vi "ProjectPaths.vi"(7 "Item":T1, 8 "Error In":errorcluster) -> (0 "Error Out":errorcluster, 3 "Path":path)   [LabVIEW 2019, in "Tools.lvlib"]
uses:
  Tools.lvlib
  ProjectPaths.ctl
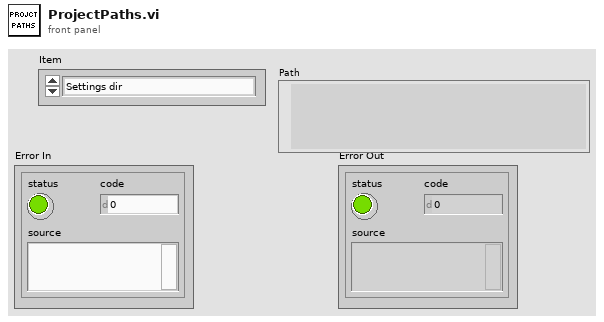
[diagram p1: front panel]
types:
  T1 = typedef "Tools.lvlib/ProjectPaths.ctl" = enum16{"Settings dir", "Logs dir", "Resources dir", "Verification file", "Users file", "Root dir"}
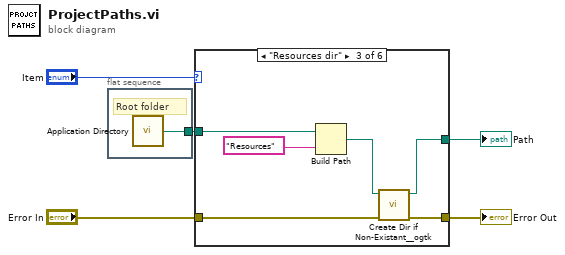
[diagram p0: block diagram]
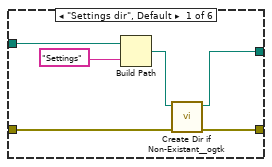
[diagram p2: hidden frame]
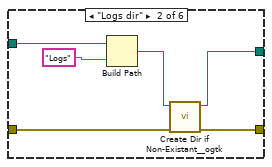
[diagram p3: hidden frame]
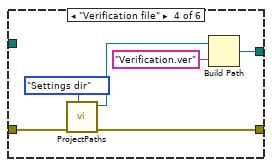
[diagram p4: hidden frame]
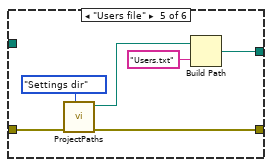
[diagram p5: hidden frame]
diagram:
  n1 = flat-sequence {
    tunnel: [w6] -> w4
    frame #0 {
      # "Root folder"
      n2 = call <vilib>:"Application Directory.vi"() -> ("Application Directory"=w6:path)
    }
  }
  n3 = case shown="\"Resources dir\"" "Item" {
    tunnel: w4 -> [w11 w18 w24 _ _ w38]
    tunnel: [w7 w13 w19 w26 w32 w38] -> w1
    tunnel: [w9 w15 w21 w29 w35 w37] -> w2
    tunnel: "Error In" -> [w10 w16 w22 w30 w36 w37]
    frame "Settings dir", Default {
      n4 = Build Path(base path=w11, name or relative path="Settings") -> (appended path=w8:path)
      n5 = call <userlib>:"Create Dir if Non-Existant__ogtk.vi"("error in (no error)"=w10, "Directory Path"=w8) -> ("error out"=w9:errorcluster, "dup Directory Path"=w7:path)  [unwired: 7 in, 1 out]
    }
    frame "Logs dir" {
      n6 = Build Path(base path=w18, name or relative path="Logs") -> (appended path=w14:path)
      n7 = call <userlib>:"Create Dir if Non-Existant__ogtk.vi"("error in (no error)"=w16, "Directory Path"=w14) -> ("error out"=w15:errorcluster, "dup Directory Path"=w13:path)  [unwired: 7 in, 1 out]
    }
    frame "Resources dir" {
      n8 = Build Path(base path=w24, name or relative path="Resources") -> (appended path=w20:path)
      n9 = call <userlib>:"Create Dir if Non-Existant__ogtk.vi"("error in (no error)"=w22, "Directory Path"=w20) -> ("error out"=w21:errorcluster, "dup Directory Path"=w19:path)  [unwired: 7 in, 1 out]
    }
    frame "Verification file" {
      n10 = call "ProjectPaths.vi"("Item"=ProjectPaths."Settings dir", "Error In"=w30) -> ("Error Out"=w29:errorcluster, "Path"=w27:path)  [unwired: 8 in]
      n11 = Build Path(base path=w27, name or relative path="Verification.ver") -> (appended path=w26:path)
    }
    frame "Users file" {
      n12 = call "ProjectPaths.vi"("Item"=ProjectPaths."Settings dir", "Error In"=w36) -> ("Error Out"=w35:errorcluster, "Path"=w33:path)  [unwired: 8 in]
      n13 = Build Path(base path=w33, name or relative path="Users.txt") -> (appended path=w32:path)
    }
    frame "Root dir" {
    }
  }
  "Error Out" <- w2
  "Path" <- w1
